vi "Post-Build Action.vi"(5 "Files Generated by Build":path[](array[path]), 6 "Top Level/Always Included VIs":path[](array[path]), 7 "Destination Path":path, 8 "error in (no error)":errorcluster, 9 "Target Name":string, 10 "Build Specification Name":string, 11 "Project Path":path) -> (0 "error out":errorcluster)   [LabVIEW 2014]
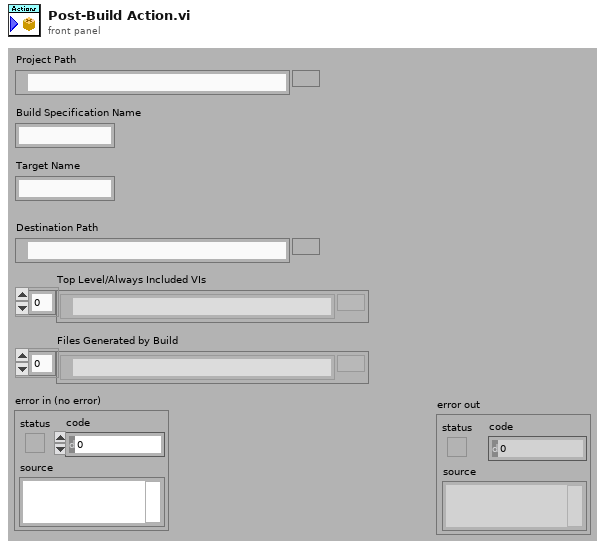
[diagram p1: front panel]
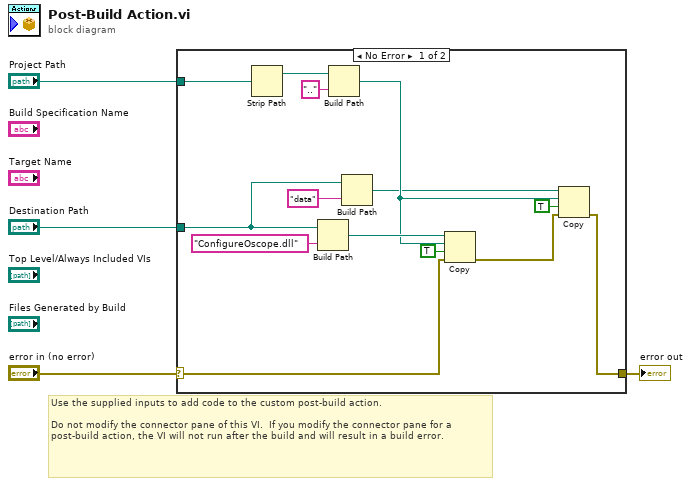
[diagram p0: block diagram]
diagram:
  # "Use the supplied inputs to add code to the custom post-build action.\n\nDo not modify the connector pane of this VI.  If you modify the connector pane for a post-build action, the VI will not run after the build and will result in a build error."
  n1 = case shown="No Error" "error in (no error)" {
    selector: "error in (no error)" -> [w12 w19]
    tunnel: "Project Path" -> [w18 _]
    tunnel: [w11 w19] -> w2
    tunnel: "Destination Path" -> [w5 _]
    frame No Error {
      n2 = Strip Path(path=w18) -> (stripped path=w17:path)  [unwired: 1 out]
      n3 = Build Path(base path=w5, name or relative path="ConfigureOscope.dll") -> (appended path=w9:path)
      n4 = Build Path(base path=w17, name or relative path="..") -> (appended path=w8:path)
      n5 = Build Path(base path=w5, name or relative path="data") -> (appended path=w6:path)
      n6 = Copy(8:w12, 9:TRUE ("overwrite (F)"), 10:w8, 11:w9) -> (0:w13:errorcluster)  [unwired: 1 in, 2 out]
      n7 = Copy(8:w13, 9:TRUE ("overwrite (F)"), 10:w8, 11:w6) -> (0:w11:errorcluster)  [unwired: 1 in, 2 out]
    }
    frame Error {
    }
  }
  "error out" <- w2
